vi "User_Test.vi"() -> ()   [LabVIEW 2020]
uses:
  User_Manage/User_Databse/User String.ctl
  <vilib>/Utility/cursorutil.llb/Set Cursor (Icon Pict).vi
  <vilib>/measure/NI_MABase.lvlib
panel:
  in  "Title":string="XXX数据采集系统"
  out "User Info":T1
  out "Graph":waveform(dbl)(graph)
  out "Time String":string
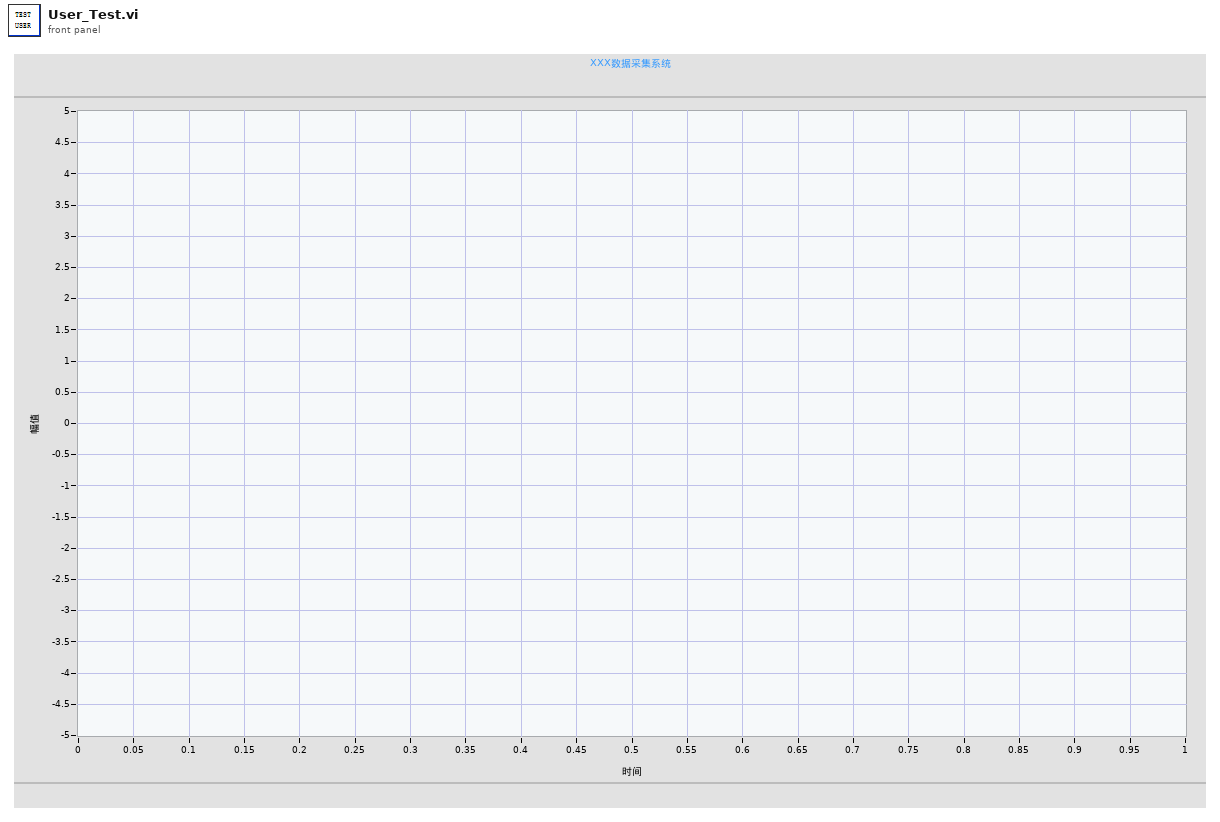
[diagram p1: front panel]
types:
  T1 = typedef "User String.ctl" = string
  T2 = typedef "User_Info.ctl" = cluster{"Name":string, "Password":string, "User_Right":u16, "Debuger?":bool, "Manager?":bool, "User_Remember_Name":bool, "User_Remember_PW":bool, "User_Right_String":string, "Null?":bool, "Language":string}
  T3 = enum32{"invalid app kind", "Development System", "Run Time System", "Student Edition", "Embedded LabVIEW", "Evaluation", "Custom"}
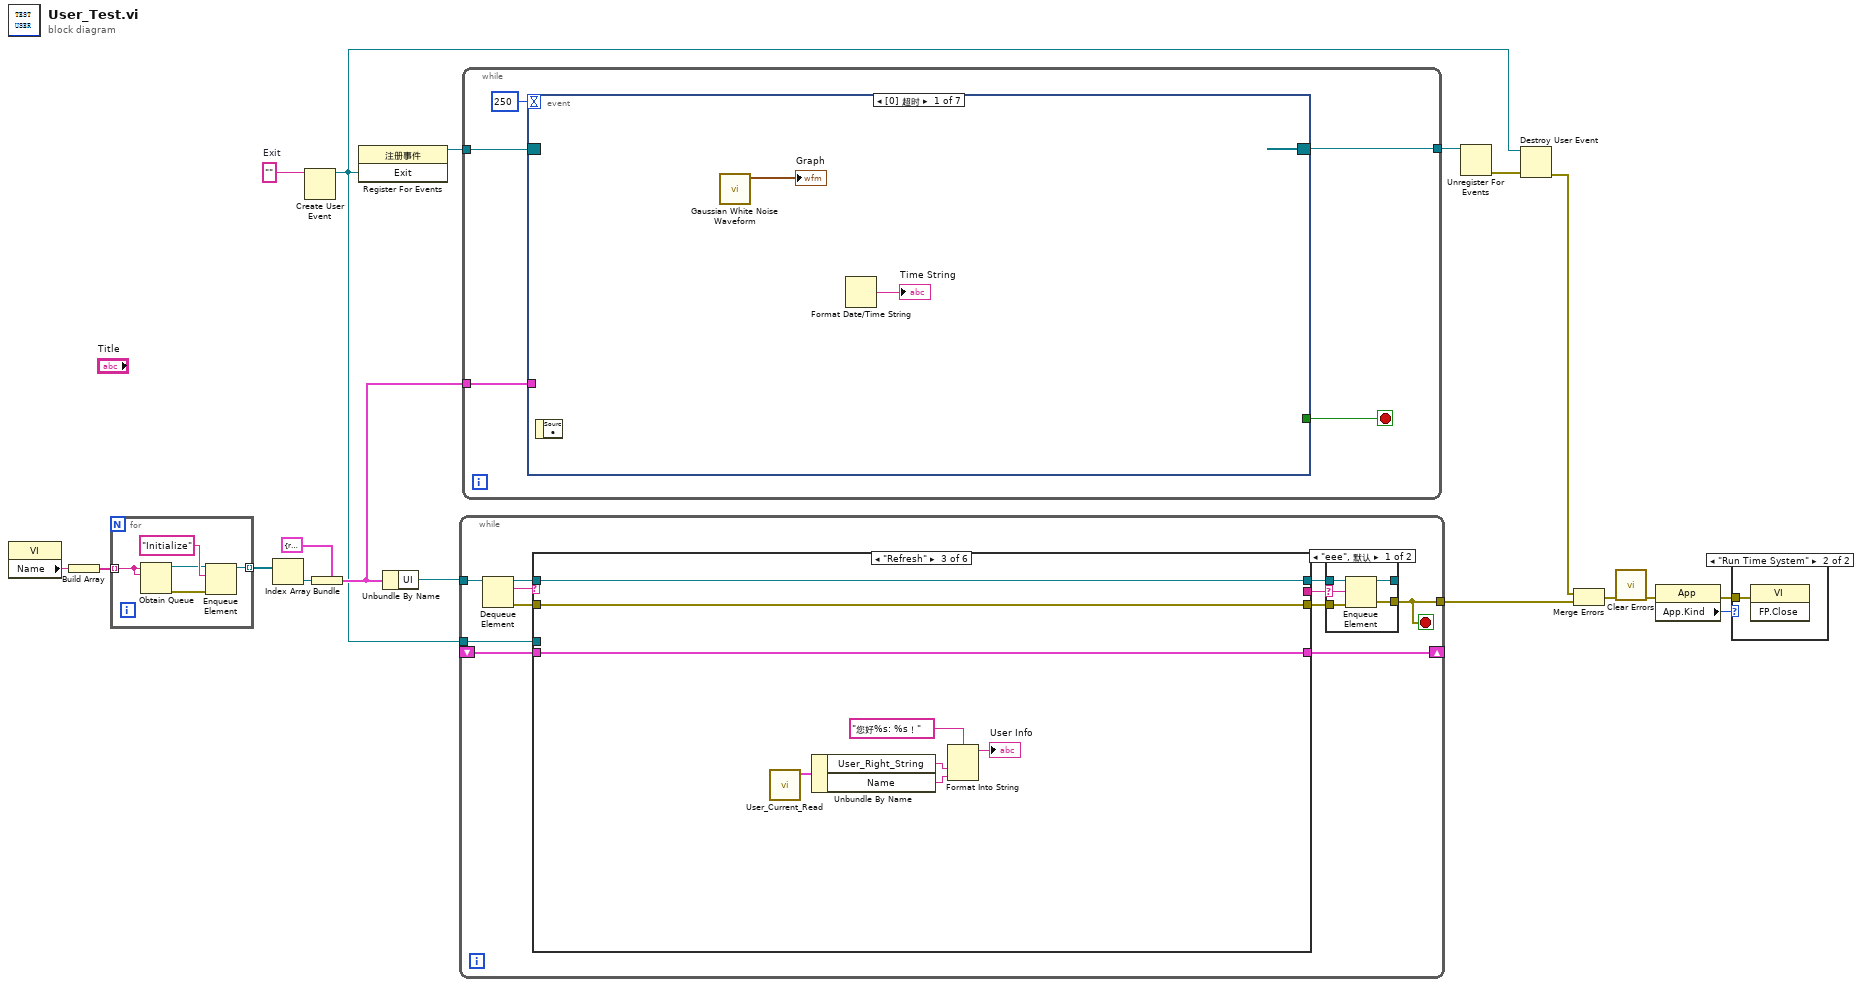
[diagram p0: block diagram]
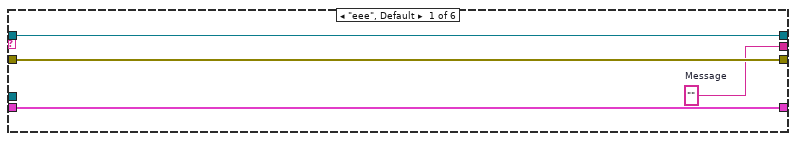
[diagram p4: hidden frame]
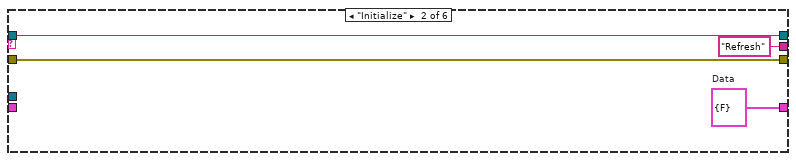
[diagram p5: hidden frame]
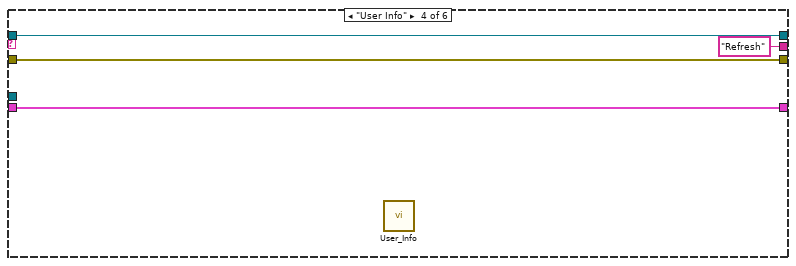
[diagram p6: hidden frame]
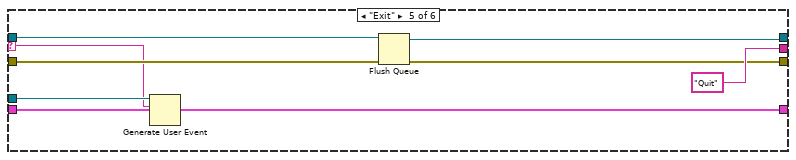
[diagram p7: hidden frame]
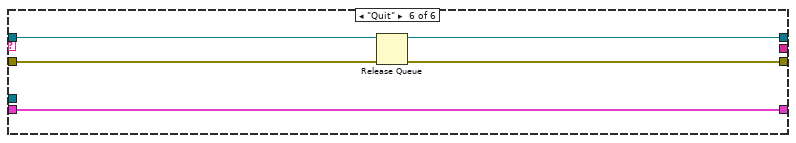
[diagram p8: hidden frame]
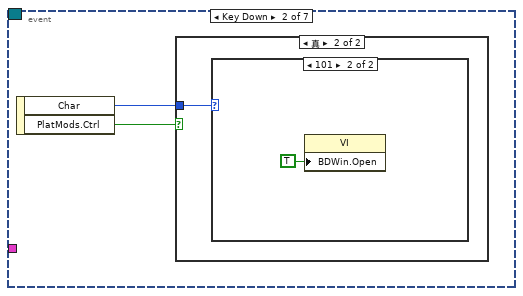
[diagram p9: hidden frame]
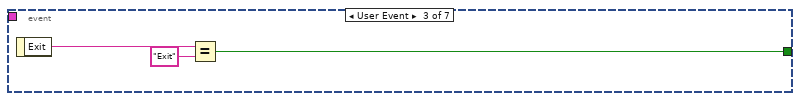
[diagram p12: hidden frame]
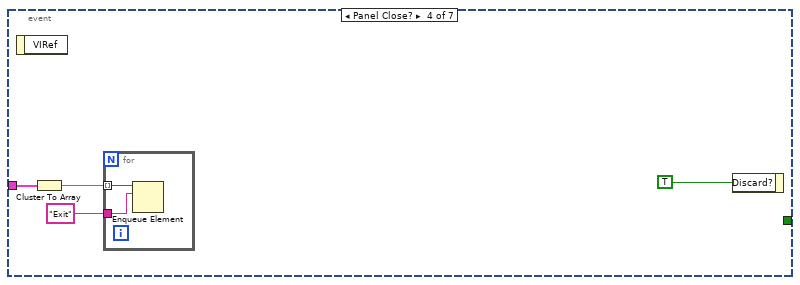
[diagram p13: hidden frame]
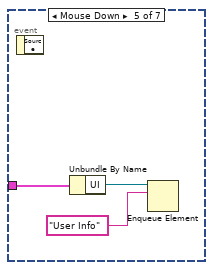
[diagram p14: hidden frame]
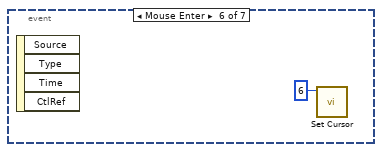
[diagram p15: hidden frame]
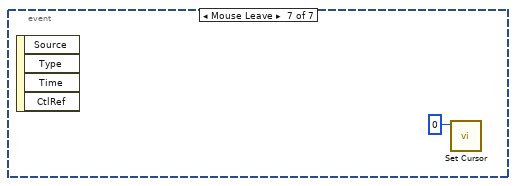
[diagram p16: hidden frame]
diagram:
  w3 = ""  # Exit
  n1 = property class="VI"() -> ("Name"=w13:string)  [unwired: 2 in, 2 out]
  n2 = Build Array(w13) -> (w14:string[])
  n3 = for {
    tunnel: w14 -> [w19] mode=indexing
    tunnel: [w20] -> w8 mode=indexing
    n4 = Obtain Queue(name (unnamed)=w19, element data type=w19) -> (queue out=w22:refnum<queue>, error out=w21:errorcluster)  [unwired: 3 in, 1 out]
    n5 = Enqueue Element(queue=w22, element="Initialize" ("元素"), error in (no error)=w21) -> (queue out=w20:refnum<queue>)  [unwired: 1 in, 2 out]
  }
  n6 = Index Array(array=w8) -> (element=w11:refnum<queue>)  [unwired: 1 in]
  n7 = Create User Event(user event datatype=w3) -> (user event=w7:refnum<user-event>)  [unwired: 1 in, 1 out]
  n8 = Bundle(cluster=cluster{"UI":refnum<queue>} {"UI"=refnum}, "UI"=w11) -> (w12:cluster{"UI":refnum<queue>})
  n9 = register-events(w7) -> (reference out=w4:refnum<event-registration>)  [unwired: 2 in, 1 out]
  n10 = Unbundle By Name(w12) -> ("UI"=w9:refnum<queue>)
  n11 = while {
    tunnel: w9 -> [w34]
    tunnel: [w24] -> w16
    shift-right: [w28] -> _
    shift-left: _ -> [w27]
    tunnel: w7 -> [w26]
    stop <- w24 stop-if-true
    n12 = Dequeue Element(queue=w34) -> (queue out=w33:refnum<queue>, element=w25:string, error out=w30:errorcluster)  [unwired: 2 in, 1 out]
    n13 = case shown="\"Refresh\"" w25 {
      selector: w25 -> [_ _ _ _ w62 _]
      tunnel: w33 -> [w45 w49 w57 w61 w67 w73]
      tunnel: [w45 w49 w57 w61 w66 w73] -> w32
      tunnel: [w44 w48 w56 w60 w65 w70] -> w31
      tunnel: w30 -> [w44 w48 w56 w60 w64 w72]
      tunnel: [w43 "Refresh" ("Message") _ "Refresh" ("Message") "Quit" ("Message") _] -> w29
      tunnel: [w42 w47 w55 w59 w69 w71] -> w28
      tunnel: w27 -> [w42 _ w55 w59 w69 w71]
      tunnel: w26 -> [_ _ _ _ w63 _]
      frame "eee", Default {
        w43 = ""  # Message
      }
      frame "Initialize" {
        w47 = cluster{"Data":bool} {"Data"=FALSE}  # Data
      }
      frame "Refresh" {
        n14 = call "User_Current_Read.vi"() -> ("User_Info"=w54:T2)  [unwired: 10 in, 1 out]
        n15 = Unbundle By Name(w54) -> ("User_Right_String"=w53:string, "Name"=w52:string)
        n16 = Format Into String(format string="您好%s: %s！" ("格式字符串"), w53, w52) -> (resulting string=→"User Info":string)  [unwired: 2 in, 1 out]
      }
      frame "User Info" {
        n17 = call "User_Info.vi"() -> ()  [unwired: 12 in]
      }
      frame "Exit" {
        n18 = Generate User Event(user event=w63, event data cluster=w62) -> ()  [unwired: 2 in, 2 out]
        n19 = Flush Queue(queue=w67, error in (no error)=w64) -> (queue out=w66:refnum<queue>, error out=w65:errorcluster)  [unwired: 1 out]
      }
      frame "Quit" {
        n20 = Release Queue(queue=w73, error in (no error)=w72) -> (error out=w70:errorcluster)  [unwired: 1 in, 2 out]
      }
    }
    n21 = case shown="\"eee\", 默认" w29 {
      selector: w29 -> [w35 _]
      tunnel: w32 -> [w39 w41]
      tunnel: w31 -> [w38 w40]
      tunnel: [w37 w40] -> w24
      tunnel: [w36 w41] -> _
      frame "eee", Default {
        n22 = Enqueue Element(queue=w39, element=w35, error in (no error)=w38) -> (queue out=w36:refnum<queue>, error out=w37:errorcluster)  [unwired: 1 in, 1 out]
      }
      frame "" {
      }
    }
  }
  n23 = while {
    tunnel: w4 -> [w77]
    tunnel: [w76] -> w6
    tunnel: w12 -> [w75]
    stop <- w78 stop-if-true
    n24 = event shown="[0] 超时" {
      selector: w77 -> [_ _ _ _ _ _ _]
      dyn-events: [_ _ _ _ _ _ _] -> w76
      timeout: 250 -> [_ _ _ _ _ _ _]
      tunnel: [_ _ w86 _ _ _ _] -> w78
      tunnel: w75 -> [_ _ _ w90 w96 _ _]
      event Timeout {
        n25 = event-data() -> ()  [unwired: 1 in, 1 out]
        n26 = call <vilib>:"Gaussian White Noise Waveform.vi"() -> ("signal out"=→"Graph":waveform(dbl))  [unwired: 10 in, 1 out]
        n27 = Format Date/Time String() -> (date/time string=→"Time String":string)  [unwired: 3 in]
      }
      event Key Down {
        n28 = event-data() -> ("Char"=w81:i16, "PlatMods.Ctrl"=w82:bool)  [unwired: 1 in]
        n29 = case shown="真" w82 {
          tunnel: w81 -> [_ w83]
          frame False {
          }
          frame True {
            n30 = case shown="101" w83 {
              frame 0, Default {
              }
              frame 101 {
                n31 = property class="VI"("BDWin.Open"=TRUE ("程序框图窗口:打开")) -> ()  [unwired: 2 in, 2 out]
              }
            }
          }
        }
      }
      event User Event {
        n32 = event-data() -> ("Exit"=w87:string)  [unwired: 1 in]
        n33 = Equal?(x=w87, y="Exit") -> (x = y?=w86:bool)
      }
      event Panel Close? {
        n34 = event-data() -> ()  [unwired: 1 in, 1 out]
        n35 = Cluster To Array(cluster=w90) -> (array=w89:refnum<queue>[])
        n36 = for {
          tunnel: w89 -> [w93] mode=indexing
          tunnel: "Exit" ("元素") -> [w92]
          n37 = Enqueue Element(queue=w93, element=w92) -> ()  [unwired: 2 in, 3 out]
        }
        n38 = event-data("Discard?"=TRUE ("放弃？")) -> ()  [unwired: 1 in, 1 out]
      }
      event Mouse Down {
        n39 = event-data() -> ()  [unwired: 1 in, 1 out]
        n40 = Unbundle By Name(w96) -> ("UI"=w95:refnum<queue>)
        n41 = Enqueue Element(queue=w95, element="User Info" ("元素")) -> ()  [unwired: 2 in, 3 out]
      }
      event Mouse Enter {
        n42 = event-data() -> ()  [unwired: 1 in, 4 out]
        n43 = call-poly <vilib>:"Set Cursor.vi"("icon"=u16 6) -> ()  [unwired: 9 in, 2 out]
      }
      event Mouse Leave {
        n44 = event-data() -> ()  [unwired: 1 in, 4 out]
        n45 = call-poly <vilib>:"Set Cursor.vi"("icon"=u16 0) -> ()  [unwired: 9 in, 2 out]
      }
    }
  }
  n46 = Unregister For Events(event registration refnum=w6) -> (error out=w5:errorcluster)  [unwired: 1 in]
  n47 = Destroy User Event(user event=w7, error in=w5) -> (error out=w15:errorcluster)
  n48 = Merge Errors(w15, w16) -> (w17:errorcluster)
  n49 = call <vilib>:"Clear Errors.vi"("error in (no error)"=w17) -> ("error out"=w18:errorcluster)  [unwired: 5 in, 1 out]
  n50 = property class="App"(error in=w18) -> (error out=w1:errorcluster, "App.Kind"=w2:T3)  [unwired: 1 in, 1 out]
  n51 = case shown="\"Run Time System\"" w2 {
    tunnel: w1 -> [_ w99]
    frame "invalid app kind", Default {
    }
    frame "Run Time System" {
      n52 = invoke class="VI" method="FP.Close"(error in=w99) -> ()  [unwired: 2 in, 3 out]
    }
  }
